vi "13.Servo project_0.vi"() -> ()   [LabVIEW 2015]
uses:
  <vilib>/myRIO/Common/Instrument Driver Framework/myRIO v1.0/PWM/vis/myRIO v1.1 Open PWM.vi
  <vilib>/myRIO/Common/Instrument Driver Framework/myRIO v1.0/UART/vis/myRIO v1.0 Close UART.vi
  <vilib>/myRIO/Common/Instrument Driver Framework/Utilities/vis/Validate Channels.vi
  <vilib>/myRIO/Common/Instrument Driver Framework/myRIO v1.0/PWM/vis/myRIO v1.0 Reserve PWM.vi
  <vilib>/myRIO/Common/Instrument Driver Framework/myRIO v1.0/PWM/vis/myRIO v1.0 Build MUX Configuration PWM.vi
  <vilib>/myRIO/Common/Instrument Driver Framework/myRIO v1.0/Resource Manager/vis/myRIO v1.0 Reserve Channel List.vi
  <vilib>/myRIO/Common/Instrument Driver Framework/myRIO v1.0/Resource Manager/vis/myRIO v1.0 Create Configuration List.vi
  <vilib>/myRIO/Common/Instrument Driver Framework/myRIO v1.0/Resource Manager/vis/myRIO v1.0 Reserve Channel.vi
  <vilib>/myRIO/Common/Instrument Driver Framework/myRIO v1.0/Resource Manager/vis/myRIO v1.0 Unreserve Channel.vi
  <vilib>/myRIO/Common/Instrument Driver Framework/myRIO v1.0/Resource Manager/vis/myRIO v1.0 Build Mutex Name.vi
  <vilib>/Utility/VariantDataType/GetNumericInfo.vi
  <vilib>/Utility/error.llb/Error Cluster From Error Code.vi
  <vilib>/myRIO/Common/Instrument Driver Framework/myRIO v1.0/myRIO v1.1 Open.vi
  <vilib>/myRIO/Common/Instrument Driver Framework/Utilities/vis/IO Manager.vi
  <vilib>/myRIO/Common/Instrument Driver Framework/Utilities/vis/Configuration Manager.vi
  <vilib>/myRIO/Common/Instrument Driver Framework/myRIO v1.0/Resource Manager/vis/myRIO v1.0 Configure IO.vi
  <vilib>/myRIO/Common/Instrument Driver Framework/myRIO v1.0/myRIO v1.0 Close.vi
  <vilib>/myRIO/Common/Instrument Driver Framework/myRIO v1.0/PWM/vis/myRIO v1.0 Write PWM.vi
  <vilib>/myRIO/Common/Instrument Driver Framework/Utilities/vis/FPGA Ref Manager.vi
  <vilib>/myRIO/Common/Instrument Driver Framework/myRIO v1.0/myRIO v1.0 Reset FPGA.vi
  <vilib>/myRIO/Common/Instrument Driver Framework/myRIO v1.0/IRQ/vis/myRIO v1.0 IRQ Info FGV.vi
  <vilib>/myRIO/Common/Instrument Driver Framework/myRIO v1.0/IRQ/vis/myRIO v1.0 Timer IRQ Info FGV.vi
  <vilib>/myRIO/Common/Instrument Driver Framework/myRIO v1.0/IRQ/vis/myRIO v1.0 ISR Agent.vi
  <vilib>/myRIO/Instrument Drivers/Utilities/Utilities.lvlib
  <vilib>/myRIO/Instrument Drivers/Onboard IO/PWM/PWM.lvlib
panel:
  in  "Tab Control 2":enum32{"Page 1", "Page 2"}(tab)
  out "offset [%FS] 2":dbl
  in  "null offset 2":bool
  out "duty cycle [%] 2":dbl
  out "pulse width [ms] 2":dbl=1.5
  in  "freq [Hz] 2":dbl=50.0
  in  "?":dbl(slide) scale=-100.0..50.0
  in  "PWM channel 2":tag="B/PWM0"
  in  "[ESC] 2":bool
  out "offset [%FS] 3":dbl
  in  "null offset 3":bool
  out "duty cycle [%] 3":dbl
  out "pulse width [ms] 3":dbl=1.5
  in  "freq [Hz] 3":dbl=50.0
  in  "?":dbl(slide) scale=-100.0..50.0
  in  "[ESC] 3":bool
  in  "PWM channel 3":tag="B/PWM0"
  out "offset [%FS] 4":dbl
  in  "null offset 4":bool
  out "duty cycle [%] 4":dbl
  out "pulse width [ms] 4":dbl=1.5
  in  "freq [Hz] 4":dbl=50.0
  in  "?":dbl(slide) scale=-100.0..-50.0
  in  "[ESC] 4":bool
  in  "PWM channel 4":tag="B/PWM0"
  # "Rotation left right"
  # "Rotation upper and down"
  # "any object pic"
  # "27"
  # "Pardeep kumar"
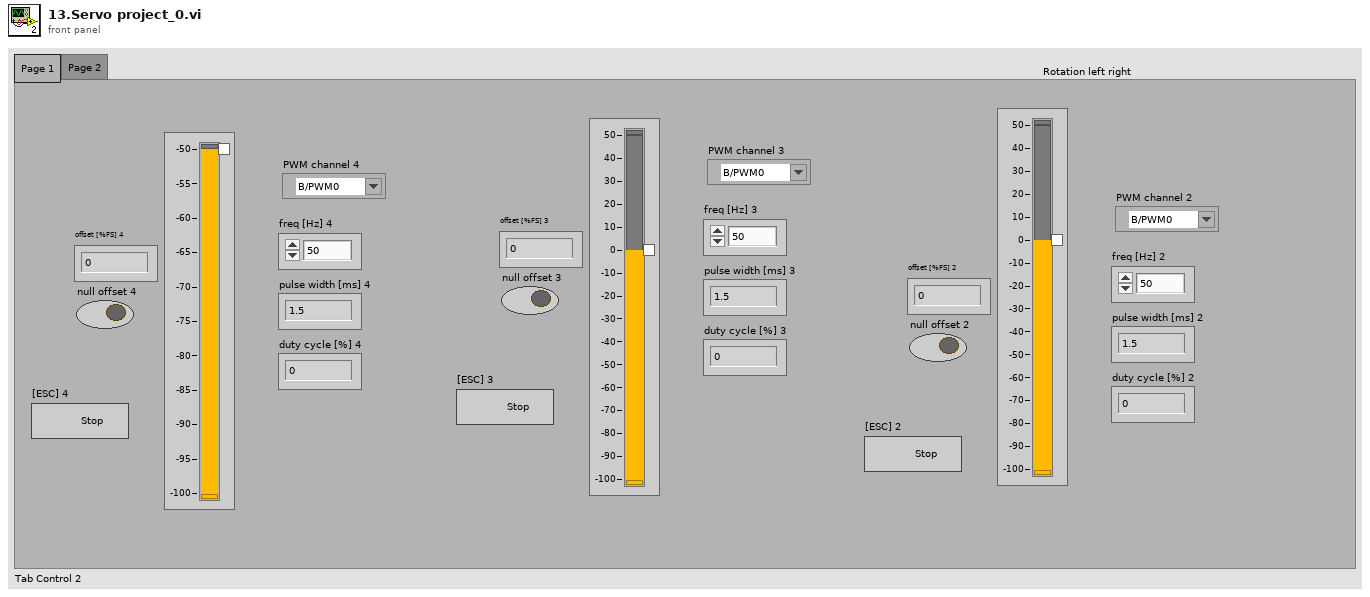
[diagram p1: front panel]
types:
  T1 = typedef "PWM.lvlib/PWM Reference.ctl" = cluster{"myRIO Reference":T2, "PWM Channels Enum":T6, "PWM Configuration":T7}
  T2 = typedef "myRIO Generic Hardware Reference.ctl" = cluster{"myRIO Model":T3, "myRIO Hardware Reference":T4}
  T3 = typedef "Hardware Version Enum.ctl" = enum16{"Unknown", "myRIO-1900", "myRIO-1950", "roboRIO"}
  T4 = typedef "myRIO v1.0 Reference.ctl" = cluster{"Generic FPGA Reference":T5, "Allow multiple opens":bool}
  T5 = typedef "Generic FPGA Reference.ctl" = refnum<k20>
  T6 = typedef "PWM Channels Enum.ctl" = enum16{"Not Connected", "C/PWM0", "C/PWM1", "A/PWM0", "A/PWM1", "A/PWM2", "B/PWM0", "B/PWM1", "B/PWM2", "PWM/PWM0", "PWM/PWM1", "PWM/PWM2", "PWM/PWM3", "PWM/PWM4", "PWM/PWM5", "PWM/PWM6", "PWM/PWM7", "PWM/PWM8", "PWM/PWM9"}
  T7 = typedef "PWM.lvlib/PWM Configuration.ctl" = cluster{"Frequency":dbl, "Duty Cycle":dbl}
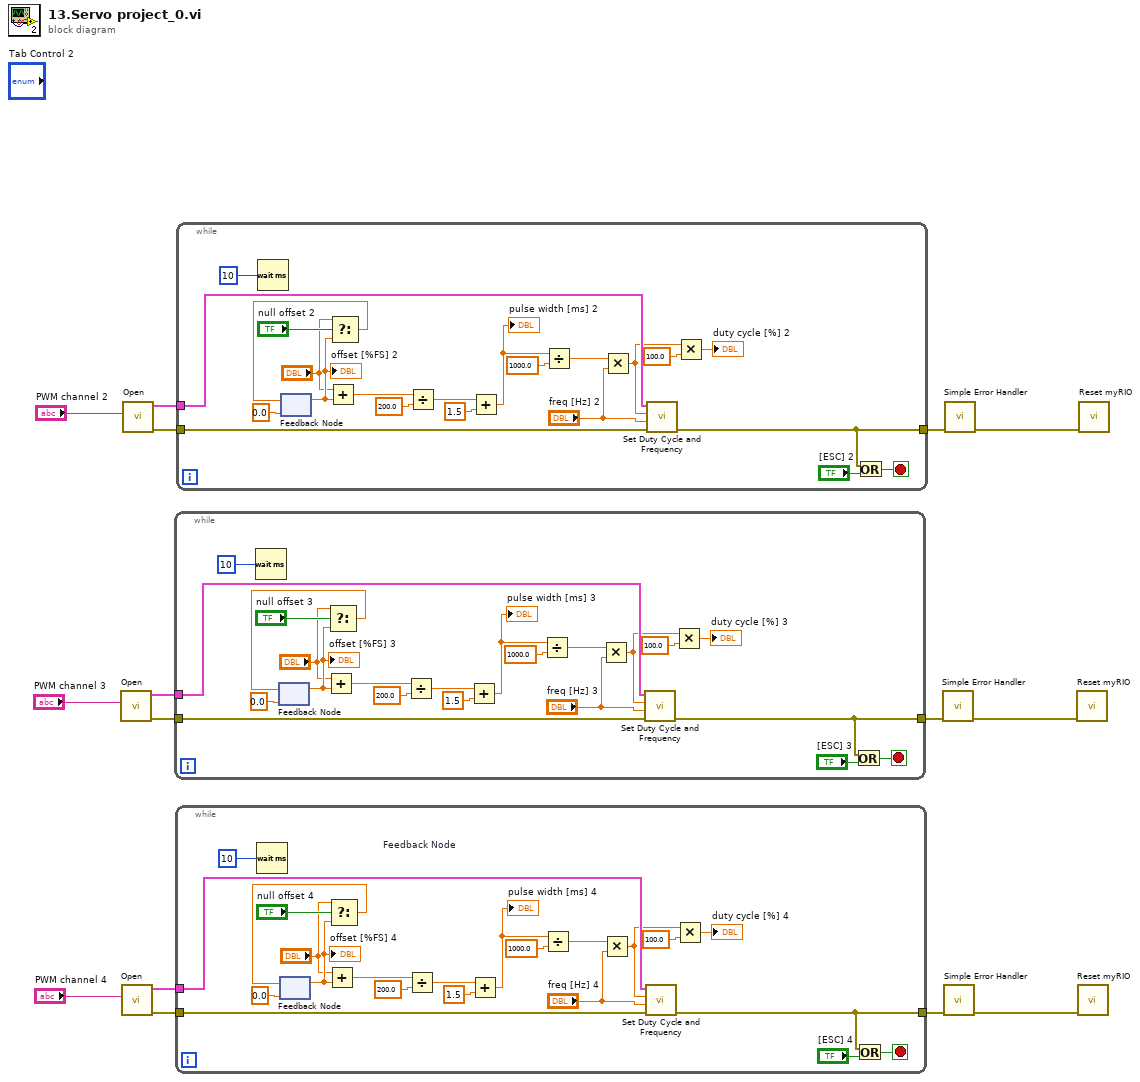
[diagram p0: block diagram]
diagram:
  n1 = call <vilib>:"Open.vi"("Channel Name"="PWM channel 3") -> ("error out"=w7:errorcluster, "PWM Ref Out"=w8:T1)  [unwired: 9 in]
  n2 = call <vilib>:"Open.vi"("Channel Name"="PWM channel 4") -> ("error out"=w2:errorcluster, "PWM Ref Out"=w3:T1)  [unwired: 9 in]
  n3 = call <vilib>:"Open.vi"("Channel Name"="PWM channel 2") -> ("error out"=w12:errorcluster, "PWM Ref Out"=w13:T1)  [unwired: 9 in]
  n4 = while {
    tunnel: w8 -> [w29]
    tunnel: w7 -> [w28]
    tunnel: [w26] -> w6
    stop <- w37 stop-if-true
    n5 = Wait (ms)(milliseconds to wait=u32 10) -> ()  [unwired: 1 out]
    n6 = feedback #1 "Feedback Node"(0.0 ("position [%FS]")) -> (w22:dbl)
    "offset [%FS] 3" <- w22
    n7 = Add(x="?", y=w22) -> (x+y=w23:dbl)
    n8 = Select(t="?", s="null offset 3", f=w22) -> (s? t:f=w24:dbl)
    n9 = feedback-in #1(w24) -> ()
    n10 = Divide(x=w23, y=200.0) -> (x/y=w33:dbl)
    n11 = Add(x=w33, y=1.5) -> (x+y=w31:dbl)
    "pulse width [ms] 3" <- w31
    n12 = Divide(x=w31, y=1000.0) -> (x/y=w20:dbl)
    n13 = Multiply(x=w20, y="freq [Hz] 3") -> (x*y=w17:dbl)
    n14 = call <vilib>:"Set Duty Cycle and Frequency.vi"("error in (no error)"=w28, "Frequency [Hz]"="freq [Hz] 3", "Duty Cycle"=w17, "PWM Ref In"=w29) -> ("error out"=w26:errorcluster)  [unwired: 5 in, 1 out]
    n15 = Multiply(x=w17, y=100.0) -> (x*y=→"duty cycle [%] 3":dbl)
    n16 = Or(x=w26, y="[ESC] 3") -> (x .or. y?=w37:bool)
  }
  n17 = while {
    tunnel: w3 -> [w51]
    tunnel: w2 -> [w50]
    tunnel: [w48] -> w1
    stop <- w59 stop-if-true
    n18 = Wait (ms)(milliseconds to wait=u32 10) -> ()  [unwired: 1 out]
    n19 = feedback #2(0.0 ("position [%FS]")) -> (w44:dbl)
    "offset [%FS] 4" <- w44
    n20 = Add(x="?", y=w44) -> (x+y=w45:dbl)
    n21 = Select(t="?", s="null offset 4", f=w44) -> (s? t:f=w46:dbl)
    n22 = feedback-in #2(w46) -> ()
    n23 = Divide(x=w45, y=200.0) -> (x/y=w55:dbl)
    n24 = Add(x=w55, y=1.5) -> (x+y=w53:dbl)
    "pulse width [ms] 4" <- w53
    n25 = Divide(x=w53, y=1000.0) -> (x/y=w42:dbl)
    n26 = Multiply(x=w42, y="freq [Hz] 4") -> (x*y=w39:dbl)
    n27 = call <vilib>:"Set Duty Cycle and Frequency.vi"("error in (no error)"=w50, "Frequency [Hz]"="freq [Hz] 4", "Duty Cycle"=w39, "PWM Ref In"=w51) -> ("error out"=w48:errorcluster)  [unwired: 5 in, 1 out]
    n28 = Multiply(x=w39, y=100.0) -> (x*y=→"duty cycle [%] 4":dbl)
    n29 = Or(x=w48, y="[ESC] 4") -> (x .or. y?=w59:bool)
  }
  n30 = while {
    tunnel: w13 -> [w73]
    tunnel: w12 -> [w72]
    tunnel: [w70] -> w11
    stop <- w81 stop-if-true
    n31 = Wait (ms)(milliseconds to wait=u32 10) -> ()  [unwired: 1 out]
    n32 = feedback #3(0.0 ("position [%FS]")) -> (w66:dbl)
    "offset [%FS] 2" <- w66
    n33 = Add(x="?", y=w66) -> (x+y=w67:dbl)
    n34 = Select(t="?", s="null offset 2", f=w66) -> (s? t:f=w68:dbl)
    n35 = feedback-in #3(w68) -> ()
    n36 = Divide(x=w67, y=200.0) -> (x/y=w77:dbl)
    n37 = Add(x=w77, y=1.5) -> (x+y=w75:dbl)
    "pulse width [ms] 2" <- w75
    n38 = Divide(x=w75, y=1000.0) -> (x/y=w64:dbl)
    n39 = Multiply(x=w64, y="freq [Hz] 2") -> (x*y=w61:dbl)
    n40 = call <vilib>:"Set Duty Cycle and Frequency.vi"("error in (no error)"=w72, "Frequency [Hz]"="freq [Hz] 2", "Duty Cycle"=w61, "PWM Ref In"=w73) -> ("error out"=w70:errorcluster)  [unwired: 5 in, 1 out]
    n41 = Multiply(x=w61, y=100.0) -> (x*y=→"duty cycle [%] 2":dbl)
    n42 = Or(x=w70, y="[ESC] 2") -> (x .or. y?=w81:bool)
  }
  n43 = call <vilib>:"Simple Error Handler.vi"("error in (no error)"=w6) -> ("error out"=w10:errorcluster)  [unwired: 4 in, 4 out]
  n44 = call <vilib>:"Simple Error Handler.vi"("error in (no error)"=w1) -> ("error out"=w5:errorcluster)  [unwired: 4 in, 4 out]
  n45 = call <vilib>:"Simple Error Handler.vi"("error in (no error)"=w11) -> ("error out"=w15:errorcluster)  [unwired: 4 in, 4 out]
  n46 = call <vilib>:"Reset myRIO.vi"("error in (no error)"=w10) -> ()  [unwired: 10 in, 1 out]
  n47 = call <vilib>:"Reset myRIO.vi"("error in (no error)"=w5) -> ()  [unwired: 10 in, 1 out]
  n48 = call <vilib>:"Reset myRIO.vi"("error in (no error)"=w15) -> ()  [unwired: 10 in, 1 out]
